vi "Init.vi"(8 "error in (no error)":errorcluster, 11 "Domain_Steady_2D_Polygon":refnum<class "NI_Domain_Steady_2D_Polygon.lvclass">) -> (0 "error out":errorcluster, 3 "initialized Domain_Steady_2D_Polygon":refnum<class "NI_Domain_Steady_2D_Polygon.lvclass">)   [LabVIEW 2020, in "NI_PDE.lvlib" / "NI_Domain_Steady_2D_Polygon.lvclass"]
uses:
  <vilib>/gmath/pde.llb/DomainClass/Domain_Steady_2D_Polygon/NI_Domain_Steady_2D_Polygon.lvclass
  <vilib>/gmath/pde.llb/DomainClass/Class Type.ctl
  <vilib>/gmath/pde.llb/DomainClass/Domain_Steady_2D_Polygon/NI_Domain_Steady_2D_Polygon.lvclass/NI_Domain_Steady_2D_Polygon.ctl
  <vilib>/gmath/pde.llb/DomainClass/NI_Domain.lvclass
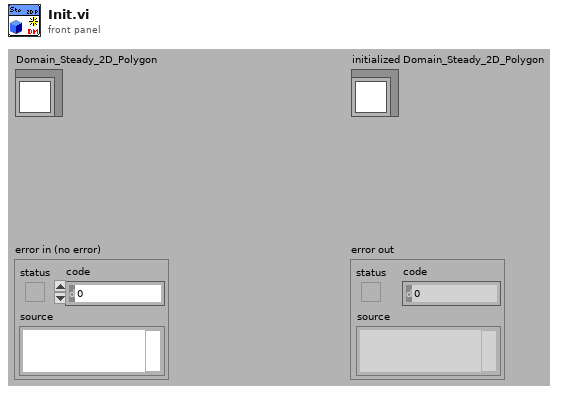
[diagram p1: front panel]
types:
  T1 = typedef "NI_PDE.lvlib/NI_Domain.lvclass/Class Type.ctl" = i32
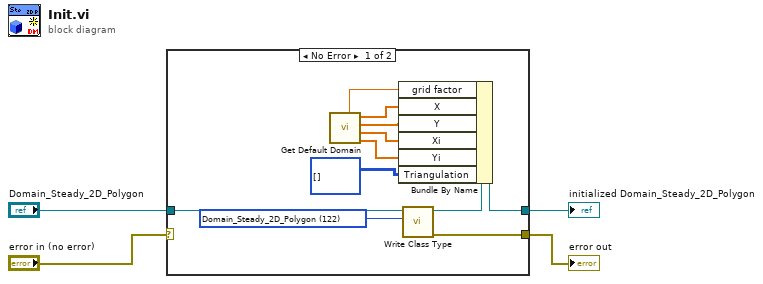
[diagram p0: block diagram]
diagram:
  n1 = case shown="No Error" "error in (no error)" {
    selector: "error in (no error)" -> [_ w17]
    tunnel: [w12 w16] -> w4
    tunnel: [w11 w17] -> w3
    tunnel: "Domain_Steady_2D_Polygon" -> [w14 w16]
    frame No Error {
      w15 = T1 122 items=["Domain"=0, "Domain_Steady"=100, "Domain_Steady_2D_Rect"=121, "Domain_Steady_2D_Polygon"=122, "Domain_Evolut"=200, "Domain_Evolut_1D"=210, "Domain_Evolut_2D_Rect"=221] ("domain class type")
      n2 = call <vilib>:"Get Default Domain.vi"() -> ("Yi"=w6:dbl[], "Xi"=w7:dbl[], "Y"=w10:dbl[], "X"=w8:dbl[], "grid factor"=w9:dbl)  [unwired: 7 out]
      n3 = call-dynamic "Write Class Type.vi"("domain class type"=w15, "Domain.lvclass in"=w14) -> ("error out"=w11:errorcluster, "Domain.lvclass out"=w13:refnum<class "NI_Domain_Steady_2D_Polygon.lvclass">)  [unwired: 1 in, 7 out]
      n4 = Bundle By Name(cluster=w13, "grid factor"=w9, "X"=w8, "Y"=w10, "Xi"=w7, "Yi"=w6, "Triangulation"=i32[][] []) -> (w12:refnum<class "NI_Domain_Steady_2D_Polygon.lvclass">)
    }
    frame Error {
    }
  }
  "initialized Domain_Steady_2D_Polygon" <- w4
  "error out" <- w3
